vi "makeTIUnderlayPlotCommands.vi"(6 "plotInfoArray":T1(array[cluster]), 9 "Scale":dbl=300.0 caption="Scale 1:" min=1.0 max=10000.0 step=50.0) -> (1 "UnderlayPlotSeries":string[](array[string]), 2 "Pre-plot Injection":string, 3 "Basics Visible":bool[](array[boolean]))   [LabVIEW 2014]
uses:
  at.ctl
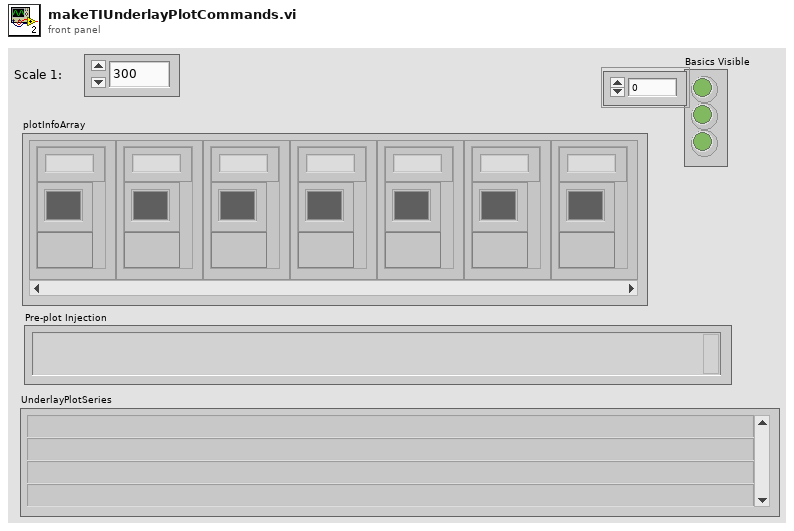
[diagram p1: front panel]
types:
  T1 = cluster{"Plot Name":string, "Plot.Plot Color":u32, "Plot.Visible?":bool}[]
  T2 = typedef "at.ctl" = cluster{"XcoordSys":string, "YcoordSys":string, "Xvalue":dbl, "Yvalue":dbl}
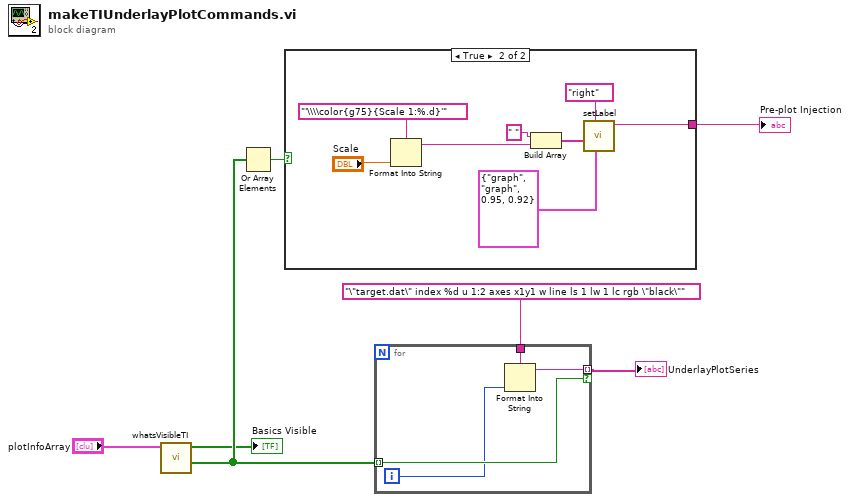
[diagram p0: block diagram]
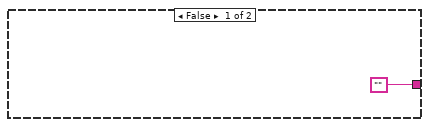
[diagram p2: hidden frame]
diagram:
  n1 = call "whatsVisibleTI.vi"("TIplotInfoArray"="plotInfoArray") -> ("Targets Visible"=w4:bool[], "Basics Visible"=→"Basics Visible":bool[])  [unwired: 9 in]
  n2 = Or Array Elements(Boolean array=w4) -> (logical OR=w2:bool)
  n3 = case shown="True" w2 {
    tunnel: ["" w9] -> w3
    frame False {
    }
    frame True {
      n4 = Format Into String(format string="'\\\\color{g75}{Scale 1:%.d}'", "Scale") -> (resulting string=w16:string)  [unwired: 2 in, 1 out]
      n5 = Build Array(" " ("element"), w16) -> (w15:string[])
      n6 = call "setLabel.vi"("\"At\" location"=T2 {"XcoordSys"="graph", "YcoordSys"="graph", "Xvalue"=0.95, "Yvalue"=0.92} ("\"At\" location"), "Justify"="right", "multilineLabel"=w15) -> ("String out"=w9:string)  [unwired: 7 in, 1 out]
    }
  }
  "Pre-plot Injection" <- w3
  n7 = for {
    tunnel: [w20] -> w5 mode=indexing if=w19
    tunnel: w4 -> [w19] mode=indexing
    tunnel: "\"target.dat\" index %d u 1:2 axes x1y1 w line ls 1 lw 1 lc rgb \"black\"" ("String") -> [w18]
    i -> [w17]
    n8 = Format Into String(format string=w18, w17) -> (resulting string=w20:string)  [unwired: 2 in, 1 out]
  }
  "UnderlayPlotSeries" <- w5
